vi "niRFUtil LCAPI Copy 1D Array (4 I32).vi"(0 "Source0 1D Array (I32)":i32[](array[numeric]), 5 "Source1 1D Array (I32)":i32[](array[numeric]), 7 "Source2 1D Array (I32)":i32[](array[numeric]), 9 "Source3 1D Array (I32)":i32[](array[numeric]), 11 "error in (no error)":errorcluster, 12 "Data Copy Descriptor":u64) -> (4 "Source0 Out":i32[](array[numeric]), 6 "Source1 Out":i32[](array[numeric]), 8 "Source2 Out":i32[](array[numeric]), 10 "Source3 Out":i32[](array[numeric]), 15 "error out":errorcluster)   [LabVIEW 2015, in "niRFUtil.lvlib"]
uses:
  niRFUtil.lvlib
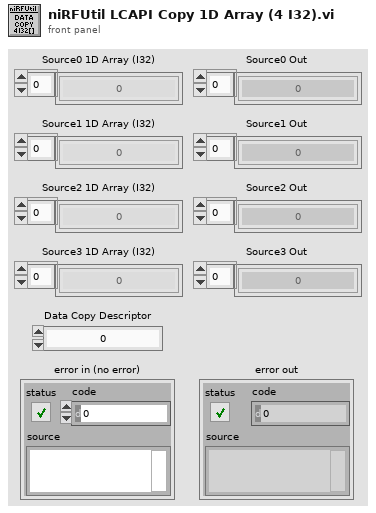
[diagram p1: front panel]
types:
  T1 = cluster{"status":bool, "return type":i32, "errorString":string}
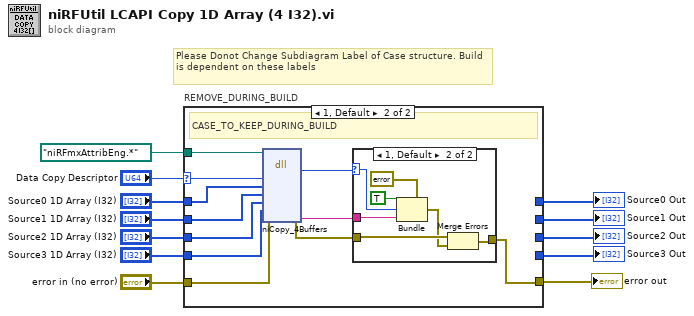
[diagram p0: block diagram]
diagram:
  # "Please Donot Change Subdiagram Label of Case structure. Build is dependent on these labels"
  n1 = case "REMOVE_DURING_BUILD" shown="1, Default" "Data Copy Descriptor" {
    selector: "Data Copy Descriptor" -> [_ w19]
    tunnel: [w17 w28] -> w12
    tunnel: "error in (no error)" -> [w17 w27]
    tunnel: "Source0 1D Array (I32)" -> [w13 w26]
    tunnel: "Source1 1D Array (I32)" -> [w14 w25]
    tunnel: "Source2 1D Array (I32)" -> [w15 w24]
    tunnel: "Source3 1D Array (I32)" -> [w16 w23]
    tunnel: [w16 _] -> w5
    tunnel: [w15 _] -> w4
    tunnel: [w14 _] -> w3
    tunnel: [w13 _] -> w2
    tunnel: path "niRFmxAttribEng.*" ("path in") -> [_ w18]
    frame 0 {
      # "Development"
    }
    frame 1, Default {
      # "CASE_TO_KEEP_DURING_BUILD"
      n2 = dll-call lib="niRFmxAttribEng.*" fn="niCopy_4Buffers"(path in=w18, error in=w27, "dataCopyDescriptor"=w19, "source0"=w26, "source1"=w25, "source2"=w24, "source3"=w23) -> (error out=w21:errorcluster, "return type"=w22:i32, "errorString"=w20:string)  [unwired: 7 in, 1 out]
      n3 = case shown="1, Default" w22 {
        selector: w22 -> [_ w34]
        tunnel: w20 -> [_ w35]
        tunnel: w21 -> [w29 w32]
        tunnel: [w29 w33] -> w28
        frame 0 {
        }
        frame 1, Default {
          n4 = Bundle(cluster=T1 {"status"=FALSE, "return type"=0, "errorString"=""}, "status"=TRUE, "return type"=w34, "errorString"=w35) -> (w31:T1)
          n5 = Merge Errors(w32, w31) -> (w33:errorcluster)
        }
      }
    }
  }
  "error out" <- w12
  "Source0 Out" <- w2
  "Source1 Out" <- w3
  "Source2 Out" <- w4
  "Source3 Out" <- w5
